vi "GetDBAL_Queue.vi"(8 "error in (no error)":errorcluster, 11 "FAMM in":refnum<class "FAMM.lvclass">) -> (0 "error out":errorcluster, 2 "DBAL-Queue":refnum<queue>, 3 "FAMM out":refnum<class "FAMM.lvclass">)   [LabVIEW 2020, in "Sgraph_lib_V1.lvlib" / "FAMM.lvclass"]
uses:
  FAMM.lvclass
  DBAL/controls/DBAL_Command.ctl
  DBAL/controls/DBAL-commands.ctl
  FAMM.lvclass/FAMM.ctl
  DBAL/DBAL.lvclass
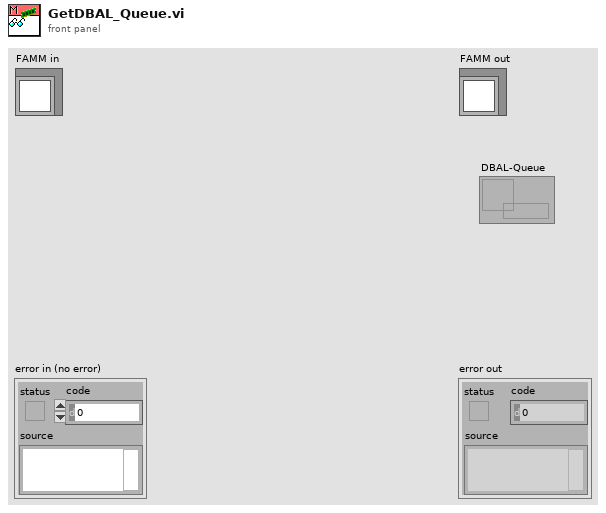
[diagram p1: front panel]
types:
  T1 = typedef "Sgraph_lib_V1.lvlib/FAMM.lvclass/FAMM-attributes.ctl" = cluster{"FAMM_PAQ_Layers":i32, "FAMM_PAQ_resolution":dbl, "PAQ_TAGs":string[], "WAQ_TAGs":string[], "EAQ_TAGs":string[], "All_TAGs":string[], "PAQtagProps":T2[], "WAQtagProps":T2[], "EAQtagProps":T2[], "DBAL_class":refnum<data-value>, "PAQ_memory":refnum<data-value>[], "PAQupdates":timestamp[], "FAMM_Size":cluster{"other":i32, "1day":i32, "1week":i32}, "DatabaseFileExtention":string, "DatabaseSaveRate":dbl, "Database_path":path, "DBAL-Queue":refnum<queue>, "OS_name":string}
  T2 = typedef "Sgraph_lib_V1.lvlib/typedef_com_TagProp.ctl" = cluster{"Description":string, "EngUnits":string, "RangeH":dbl, "RangeL":dbl, "Resolution":i32, "Obsolete":bool, "ChangeDate":timestamp, "ChangeSource":string, "ChangeReason":string, "TagFunc":u32}
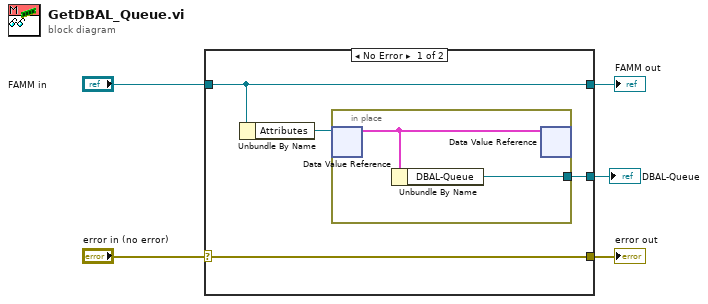
[diagram p0: block diagram]
diagram:
  n1 = case shown="No Error" "error in (no error)" {
    selector: "error in (no error)" -> [w9 w12]
    tunnel: [w9 w12] -> w4
    tunnel: [w8 w13] -> w2
    tunnel: "FAMM in" -> [w8 w13]
    tunnel: [w6 _] -> w1
    frame No Error {
      n2 = Unbundle By Name(w8) -> ("Attributes"=w7:refnum<data-value>)
      n3 = in-place {
        in-place-border: [w10] -> w6
        n4 = in-place-dvr #1(w7) -> (w11:T1)  [unwired: 1 out]
        n5 = Unbundle By Name(w11) -> ("DBAL-Queue"=w10:refnum<queue>)
        n6 = in-place-dvr #1(w11) -> ()  [unwired: 2 out]
      }
    }
    frame Error {
    }
  }
  "error out" <- w4
  "FAMM out" <- w2
  "DBAL-Queue" <- w1
